vi "TDTSyn-Register CAR Control Events.vi"(7 "Refs":refnum<vi>[](array[refnum]), 11 "error in (no error)":errorcluster) -> (8 "Event Registration Refnum":refnum<event-registration>, 15 "error out":errorcluster)   [LabVIEW 2015]
uses:
  CAR Control/Events.ctl
  CAR Control/Event Data.ctl
  CAR Control/Update Data.ctl
  CAR Control/CAR Control.xctl
panel:
  in  "temp":cluster{"Neu1":T1, "Neu2":T1, "Neu3":T1}
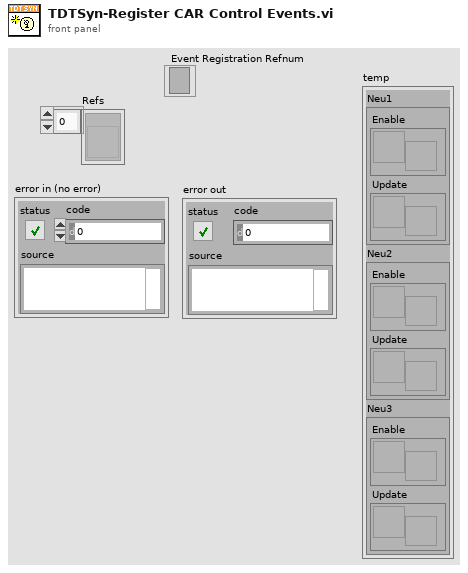
[diagram p1: front panel]
types:
  T1 = typedef "CAR Control.xctl/Events.ctl" = cluster{"Enable":refnum<user-event>, "Update":refnum<user-event>}
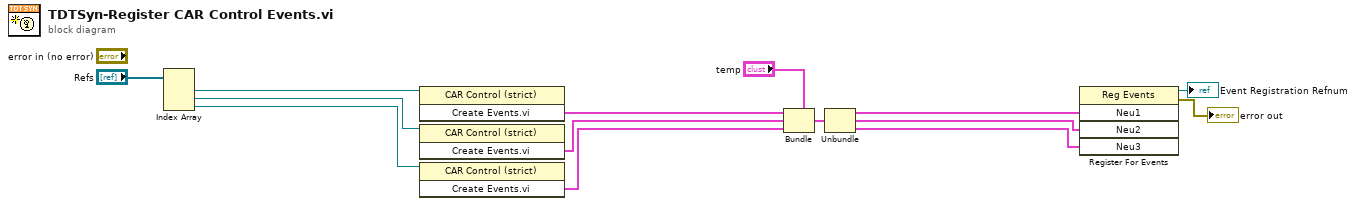
[diagram p0: block diagram]
diagram:
  n1 = Index Array(array="Refs") -> (element #1=w10:refnum<vi>, element #2=w7:refnum<vi>, element #3=w4:refnum<vi>)  [unwired: 3 in]
  n2 = invoke class="CAR Control (strict)" method="Create Events.vi"(reference=w10) -> ("Create Events.vi"=w9:T1)  [unwired: 2 in, 2 out]
  n3 = invoke class="CAR Control (strict)" method="Create Events.vi"(reference=w7) -> ("Create Events.vi"=w6:T1)  [unwired: 2 in, 2 out]
  n4 = invoke class="CAR Control (strict)" method="Create Events.vi"(reference=w4) -> ("Create Events.vi"=w3:T1)  [unwired: 2 in, 2 out]
  n5 = Bundle(cluster="temp", "Neu1"=w9, "Neu2"=w6, "Neu3"=w3) -> (w14:cluster{"Neu1":T1, "Neu2":T1, "Neu3":T1})
  n6 = Unbundle(w14) -> ("Neu1"=w8:T1, "Neu2"=w5:T1, "Neu3"=w2:T1)
  n7 = register-events(w8, w5, w2) -> (reference out=→"Event Registration Refnum":refnum<event-registration>, error out=→"error out":errorcluster)  [unwired: 2 in]
